vi "DrawToolPosition.vi"(8 "Show lines":bool, 9 "Setup":T1={"Scaling (pixels/mm)"=1.0, "Tool Diameter (inch)"=0.25, "Origin location"={"x (mm)"=10, "y (mm)"=315}, "Wood dim"={"width (inch)"=10.0, "height (inch)"=12.0}}, 10 "mouse position":cluster{"X (mm)":dbl, "Y (mm)":dbl}, 11 "dot position":cluster{"X (mm)":dbl, "Y (mm)":dbl}) -> (3 "blob":picture)   [LabVIEW 2024]
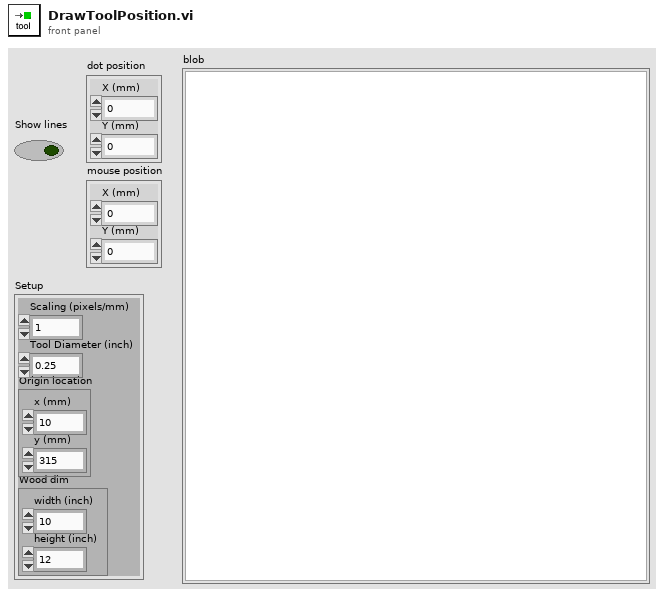
[diagram p1: front panel]
types:
  T1 = cluster{"Scaling (pixels/mm)":dbl, "Tool Diameter (inch)":dbl, "Origin location":cluster{"x (mm)":i16, "y (mm)":i16}, "Wood dim":cluster{"width (inch)":dbl, "height (inch)":dbl}}
  T2 = cluster{"Width":u16, "Style":enum32{"Solid", "Dash", "Dot", "DashDot", "DashDotDot"}}
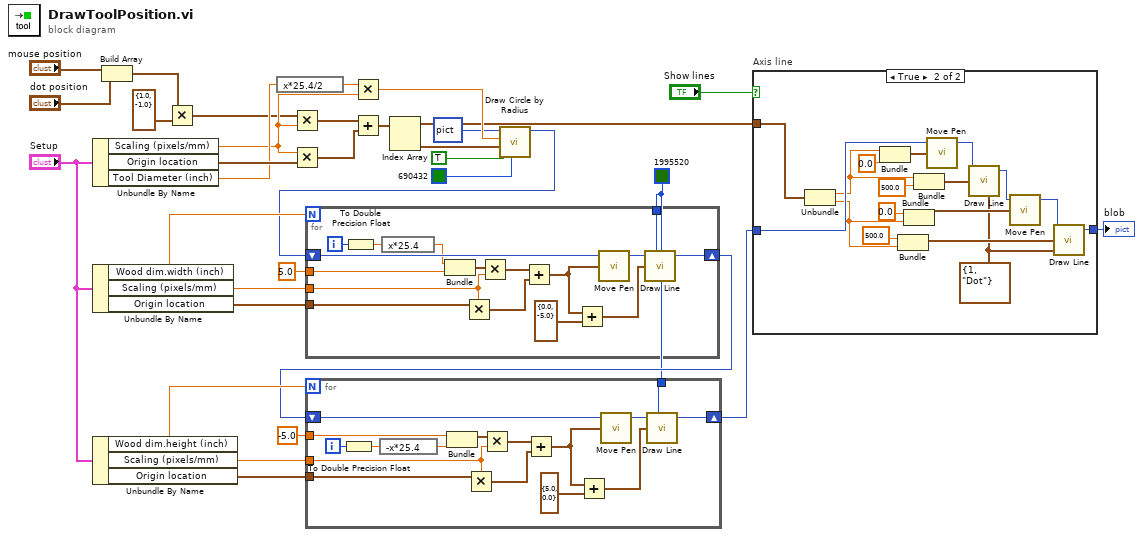
[diagram p0: block diagram]
diagram:
  w15 = u32 1995520 ("color(black)")
  n1 = Unbundle By Name("Setup") -> ("Scaling (pixels/mm)"=w27:dbl, "Origin location"=w31:cluster{"x (mm)":i16, "y (mm)":i16}, "Tool Diameter (inch)"=w29:dbl)
  n2 = Unbundle By Name("Setup") -> ("Wood dim.width (inch)"=w23:dbl, "Scaling (pixels/mm)"=w25:dbl, "Origin location"=w24:cluster{"x (mm)":i16, "y (mm)":i16})
  n3 = Unbundle By Name("Setup") -> ("Wood dim.height (inch)"=w22:dbl, "Scaling (pixels/mm)"=w20:dbl, "Origin location"=w21:cluster{"x (mm)":i16, "y (mm)":i16})
  n4 = Build Array("mouse position", "dot position") -> (w9:cluster{"X (mm)":dbl, "Y (mm)":dbl}[])
  n5 = Multiply(x=w9, y=cluster{"X":dbl, dbl} {"X"=1.0, -1.0} ("output cluster")) -> (x*y=w12:cluster{dbl, dbl}[])
  n6 = expression code="x*25.4/2"(w29) -> (w33:dbl)
  n7 = Multiply(x=w12, y=w27) -> (x*y=w30:cluster{dbl, dbl}[])
  n8 = Multiply(x=w27, y=w31) -> (x*y=w32:cluster{"x (mm)":dbl, "y (mm)":dbl})
  n9 = Multiply(x=w33, y=w27) -> (x*y=w6:dbl)
  n10 = Add(x=w30, y=w32) -> (x+y=w28:cluster{dbl, dbl}[])
  n11 = Index Array(array=w28) -> (element #1=w5:cluster{dbl, dbl}, element #2=w4:cluster{dbl, dbl})  [unwired: 2 in]
  n12 = call <vilib>:"Draw Circle by Radius.vi"("color(black)"=u32 690432, "fill?(F)"=TRUE, "pixel center"=w4, "radius"=w6, "picture"=picture data[5B]) -> ("new picture"=w3:picture)  [unwired: 6 in]
  n13 = for {
    N: w23 -> [_]
    tunnel: 5.0 -> [w46]
    tunnel: w25 -> [w43]
    tunnel: w24 -> [w44]
    shift-right: [w38] -> w17
    shift-left: w3 -> [w39]
    tunnel: w15 -> [w34]
    i -> [w37]
    n14 = To Double Precision Float(number=w37) -> (double precision float=w35:dbl)
    n15 = expression code="x*25.4"(w35) -> (w36:dbl)
    n16 = Bundle(w36, w46) -> (w45:cluster{dbl, dbl})  [unwired: 1 in]
    n17 = Multiply(x=w44, y=w43) -> (x*y=w47:cluster{"x (mm)":dbl, "y (mm)":dbl})
    n18 = Multiply(x=w45, y=w43) -> (x*y=w48:cluster{dbl, dbl})
    n19 = Add(x=w48, y=w47) -> (x+y=w42:cluster{dbl, dbl})
    n20 = Add(x=w42, y=cluster{dbl, dbl} {0.0, -5.0}) -> (x+y=w40:cluster{dbl, dbl})
    n21 = call <vilib>:"Move Pen.vi"("new position"=w42, "picture"=w39) -> ("new picture"=w49:picture)  [unwired: 3 in]
    n22 = call <vilib>:"Draw Line.vi"("picture"=w49, "end point"=w40, "color(black)"=w34) -> ("new picture"=w38:picture)  [unwired: 6 in]
  }
  n23 = for {
    N: w22 -> [_]
    tunnel: w20 -> [w61]
    tunnel: w21 -> [w62]
    shift-right: [w56] -> w16
    shift-left: w17 -> [w57]
    tunnel: -5.0 -> [w52]
    tunnel: w15 -> [w50]
    i -> [w55]
    n24 = To Double Precision Float(number=w55) -> (double precision float=w54:dbl)
    n25 = expression code="-x*25.4"(w54) -> (w53:dbl)
    n26 = Bundle(w52, w53) -> (w51:cluster{dbl, dbl})  [unwired: 1 in]
    n27 = Multiply(x=w62, y=w61) -> (x*y=w63:cluster{"x (mm)":dbl, "y (mm)":dbl})
    n28 = Multiply(x=w51, y=w61) -> (x*y=w64:cluster{dbl, dbl})
    n29 = Add(x=w64, y=w63) -> (x+y=w60:cluster{dbl, dbl})
    n30 = Add(x=w60, y=cluster{dbl, dbl} {5.0, 0.0}) -> (x+y=w58:cluster{dbl, dbl})
    n31 = call <vilib>:"Move Pen.vi"("new position"=w60, "picture"=w57) -> ("new picture"=w65:picture)  [unwired: 3 in]
    n32 = call <vilib>:"Draw Line.vi"("picture"=w65, "end point"=w58, "color(black)"=w50) -> ("new picture"=w56:picture)  [unwired: 6 in]
  }
  n33 = case "Axis line" shown="True" "Show lines" {
    tunnel: w5 -> [_ w83]
    tunnel: [w66 w68] -> w2
    tunnel: w16 -> [w66 w80]
    frame False {
    }
    frame True {
      w67 = T2 {"Width"=1, "Style"=enum."Dot"} ("pen")
      n34 = Unbundle(w83) -> (w79:dbl, w70:dbl)
      n35 = Bundle(w79, 0.0) -> (w81:cluster{dbl, dbl})  [unwired: 1 in]
      n36 = Bundle(500.0, w70) -> (w74:cluster{dbl, dbl})  [unwired: 1 in]
      n37 = Bundle(0.0, w70) -> (w73:cluster{dbl, dbl})  [unwired: 1 in]
      n38 = Bundle(w79, 500.0) -> (w77:cluster{dbl, dbl})  [unwired: 1 in]
      n39 = call <vilib>:"Move Pen.vi"("new position"=w81, "picture"=w80) -> ("new picture"=w76:picture)  [unwired: 3 in]
      n40 = call <vilib>:"Draw Line.vi"("picture"=w76, "end point"=w77, "pen"=w67) -> ("new picture"=w69:picture)  [unwired: 6 in]
      n41 = call <vilib>:"Move Pen.vi"("new position"=w73, "picture"=w69) -> ("new picture"=w75:picture)  [unwired: 3 in]
      n42 = call <vilib>:"Draw Line.vi"("picture"=w75, "end point"=w74, "pen"=w67) -> ("new picture"=w68:picture)  [unwired: 6 in]
    }
  }
  "blob" <- w2
